vi "clearRoot.vi"(8 "error in (no error)":errorcluster, 11 "BasicSortedList in":refnum<class "BasicSortedList.lvclass">) -> (0 "error out":errorcluster, 3 "BasicSortedList out":refnum<class "BasicSortedList.lvclass">)   [LabVIEW 2010, in "BasicSortedList.lvclass"]
uses:
  BasicSortedList.lvclass
  LLNode/LLNode.lvclass
  LinkedList/LinkedList.lvclass
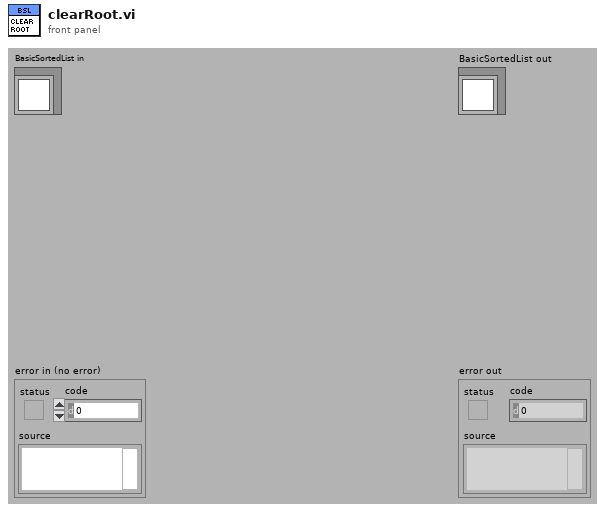
[diagram p1: front panel]
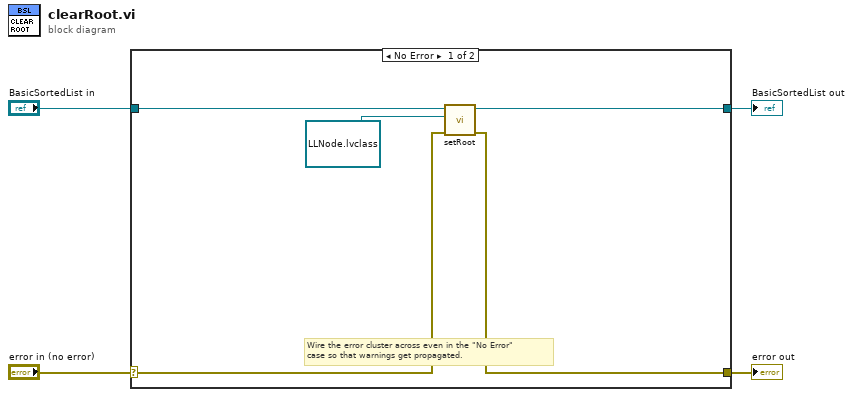
[diagram p0: block diagram]
diagram:
  n1 = case shown="No Error" "error in (no error)" {
    selector: "error in (no error)" -> [w7 w11]
    tunnel: [w6 w11] -> w3
    tunnel: [w8 w10] -> w1
    tunnel: "BasicSortedList in" -> [w9 w10]
    frame No Error {
      # "Wire the error cluster across even in the \"No Error\"\ncase so that warnings get propagated."
      n2 = call "setRoot.vi"("error in (no error)"=w7, "Root"=refnum<data-value> refnum, "LinkedList in"=w9) -> ("error out"=w6:errorcluster, "LinkedList out"=w8:refnum<class "BasicSortedList.lvclass">)  [unwired: 7 in]
    }
    frame Error {
    }
  }
  "error out" <- w3
  "BasicSortedList out" <- w1
